vi "MTM2_getSample_axialActuatorSteps.vi"(8 "error in (no error)":errorcluster, 11 "axialActuatorSteps_Ctl":T1={"private_rcvStamp"=0.0, "steps[72]"=[0, 0, 0, 0, 0, 0, 0, 0, 0, 0, 0, 0, 0, 0, 0, 0, 0, 0, 0, 0, 0, 0, 0, 0, 0, 0, 0, 0, 0, 0, 0, 0, 0, 0, 0, 0, 0, 0, 0, 0, 0, 0, 0, 0, 0, 0, 0, 0, 0, 0, 0, 0, 0, 0, 0, 0, 0, 0, 0, 0, 0, 0, 0, 0, 0, 0, 0, 0, 0, 0, 0, 0]}) -> (0 "error out":errorcluster, 2 "function return":i32, 3 "axialActuatorSteps_Ctl out":T1)   [LabVIEW 2018, in "SALLV_MTM2.lvlib"]
doc: "int MTM2_shm_getSample_axialActuatorStepsLV(MTM2_axialActuatorStepsLV *axialActuatorSteps_Ctl );"
uses:
  DataTypes/axialActuatorSteps.ctl
  SALLV_MTM2.lvlib
  SALLV_MTM2.so
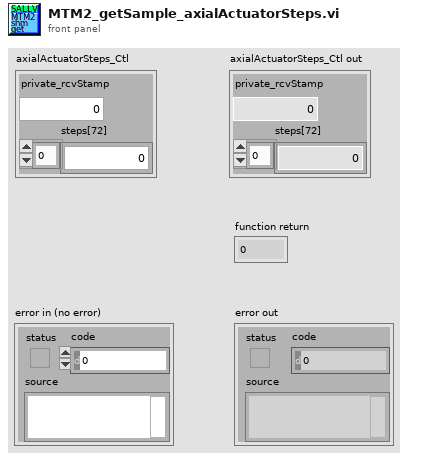
[diagram p1: front panel]
types:
  T1 = typedef "SALLV_MTM2.lvlib/axialActuatorSteps.ctl" = cluster{"private_rcvStamp":dbl, "steps[72]":i32[]}
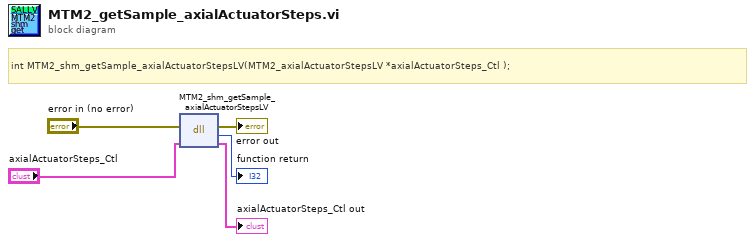
[diagram p0: block diagram]
diagram:
  # "int MTM2_shm_getSample_axialActuatorStepsLV(MTM2_axialActuatorStepsLV *axialActuatorSteps_Ctl );"
  n1 = dll-call lib="home/ttsai/Documents/salTestLabViewApi/SALLV_MTM2/SALLV_MTM2.*" fn="MTM2_shm_getSample_axialActuatorStepsLV"(error in="error in (no error)", "axialActuatorSteps_Ctl"="axialActuatorSteps_Ctl") -> (error out=→"error out":errorcluster, →"function return":i32, "axialActuatorSteps_Ctl"=→"axialActuatorSteps_Ctl out":T1)  [unwired: 2 in, 1 out]
